vi "transport image.vi"() -> ()   [LabVIEW 2019]
panel:
  out "data string":string
  out "Image 2":T1(plugin-control)
  out "Image":T1(plugin-control)
  in  "File Path":path
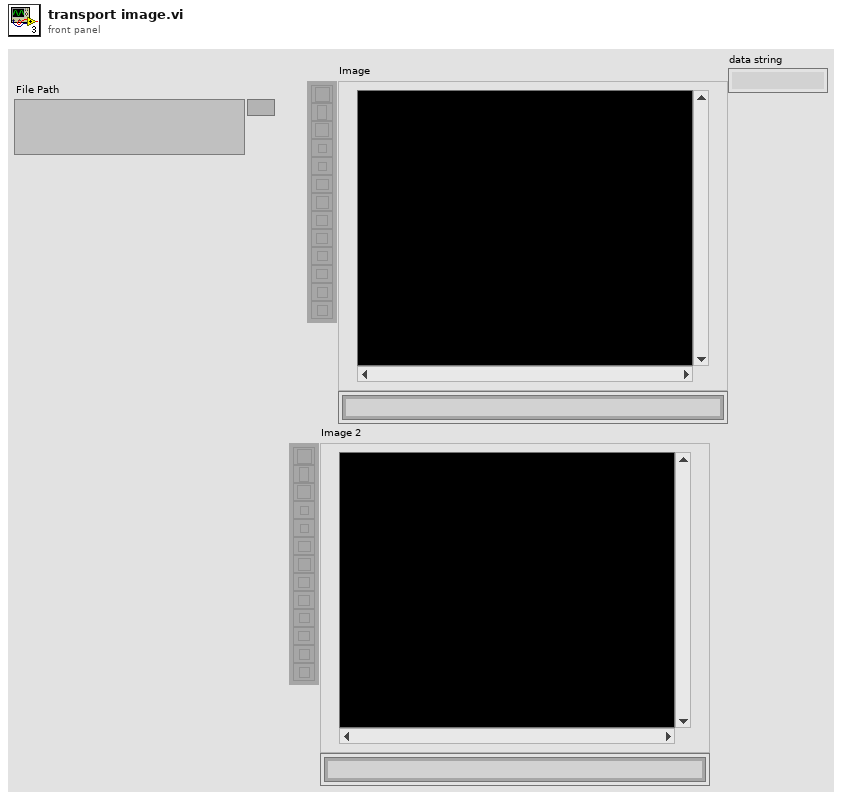
[diagram p1: front panel]
types:
  T1 = typedef "IMAQ Image.ctl" = refnum<image>
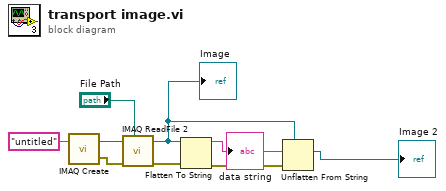
[diagram p0: block diagram]
diagram:
  n1 = call "IMAQ Create"("Image Name"="untitled") -> ("New Image"=w8:T1, "error out"=w9:errorcluster)  [unwired: 4 in]
  n2 = call "IMAQ ReadFile 2"("File Path"="File Path", "error in (no error)"=w9, "Image"=w8) -> ("error out"=w5:errorcluster, "Image Out"=w3:T1)  [unwired: 4 in, 3 out]
  "Image" <- w3
  n3 = Flatten To String(anything=w3, error in (no error)=w5) -> (data string=w1:string, error out=w4:errorcluster)  [unwired: 2 in, 1 out]
  "data string" <- w1
  n4 = Unflatten From String(type=w3, binary string=w1, error in (no error)=w4) -> (value=→"Image 2":T1)  [unwired: 2 in, 2 out]
